vi "GetDutMAC.vi"(1 "MAC模式":string, 2 "Dut_ip":string, 3 "MAC跳数":string, 4 "Client_ip":string) -> (0 "输出MAC":string)   [LabVIEW 2014]
panel:
  out "字符串":string
  out "布尔":bool=TRUE
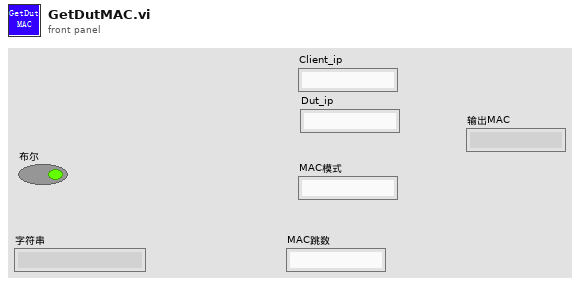
[diagram p1: front panel]
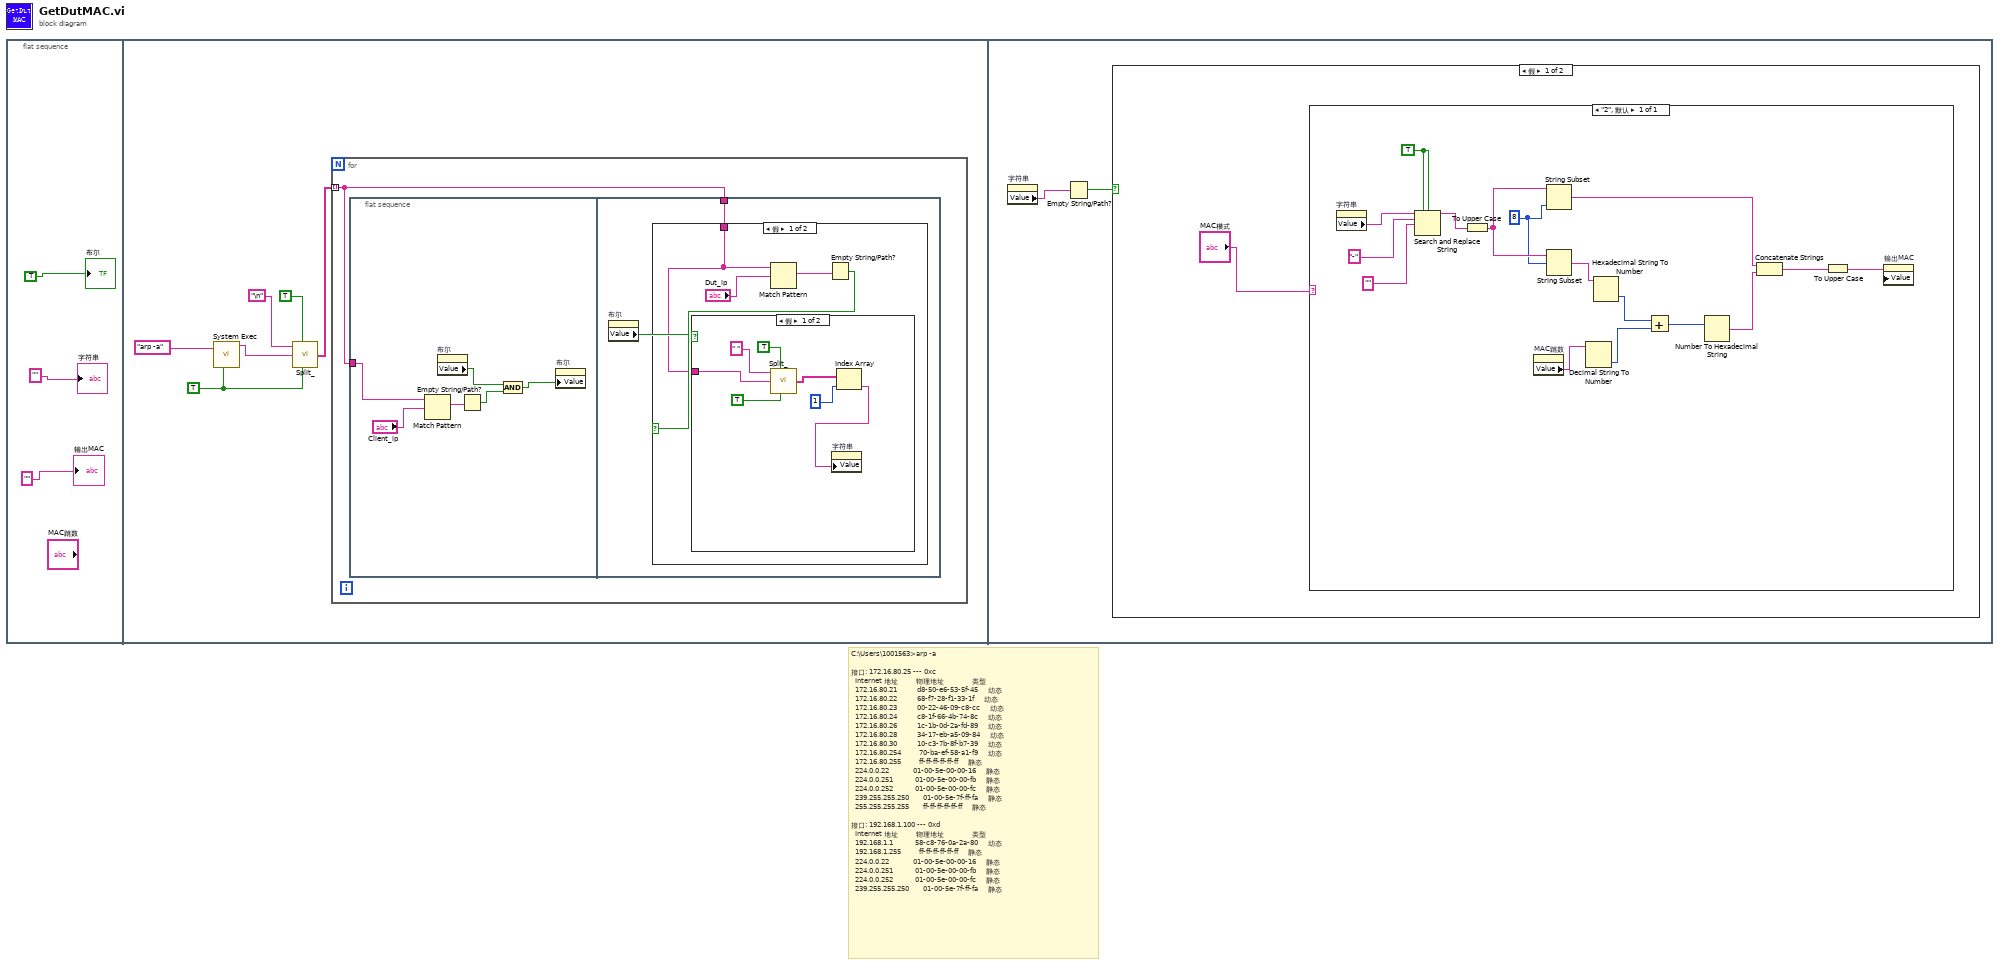
[diagram p0: block diagram]
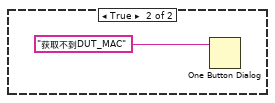
[diagram p4: hidden frame]
diagram:
  # "C:\\Users\\1001563>arp -a\n\n接口: 172.16.80.25 --- 0xc\n  Internet 地址         物理地址              类型\n  172.16.80.21          d8-50-e6-53-5f-45     动态\n  172.16.80.22          68-f7-28-f1-33-1f     动态\n  172.16.80.23          00-22-46-09-c8-cc     动态\n  172.16.80.24          c8-1f-66-4b-74-8c     动态\n  172.16.80.26          1c-1b-0d-2a-fd-89     动态\n  172.16.80.28          34-17-eb-a5-09-84     动态\n  172.16.80.30          10-c3-7b-8f-b7-39     动态\n  172.16.80.254         70-ba-ef-58-a1-f9     动态\n  172.16.80.255         ff-ff-ff-ff-ff-ff     静态\n  224.0.0.22            01-00-5e-00-00-16     静态\n  224.0.0.251           01-00-5e-00-00-fb     静态\n  224.0.0.252           01-00-5e-00-00-fc     静态\n  239.255.255.250       01-00-5e-7f-ff-fa     静态\n  255.255.255.255       ff-ff-ff-ff-ff-ff     静态\n\n接口: 192.168.1.100 --- 0xd\n  Internet 地址         物理地址              类型\n  192.168.1.1           58-c8-76-0a-2a-80     动态\n  192.168.1.255         ff-ff-ff-ff-ff-ff     静态\n  224.0.0.22            01-00-5e-00-00-16     静态\n  224.0.0.251           01-00-5e-00-00-fb     静态\n  224.0.0.252           01-00-5e-00-00-fc     静态\n  239.255.255.250       01-00-5e-7f-ff-fa     静态"
  n1 = flat-sequence {
    frame #0 {
      "布尔" <- TRUE
      "字符串" <- ""
      "输出MAC" <- ""
    }
    frame #1 {
      w5 = TRUE
      n2 = call <vilib>:"System Exec.vi"("run minimized? (F)"=w5, "command line"="arp -a") -> ("standard output"=w8:string)  [unwired: 6 in, 3 out]
      n3 = call "Split_.vi"("分隔字符串/字符(,)"="\n", "移除空字符串（T）"=TRUE, "字符串"=w8, "移除空白字符（T）"=w5) -> ("字符串数组"=w4:string[])  [unwired: 3 in]
      n4 = for {
        tunnel: w4 -> [w10] mode=indexing
        n5 = flat-sequence {
          tunnel: w10 -> [w16]
          tunnel: w10 -> [w17]
          frame #0 {
            n6 = Match Pattern(string=w16, regular expression="Client_ip") -> (match substring=w14:string)  [unwired: 1 in, 3 out]
            n7 = property on="布尔" class="Bool (严格)"() -> ("Value"=w12:bool)  [unwired: 2 in, 2 out]
            n8 = Empty String/Path?(string/path=w14) -> (empty?=w13:bool)
            n9 = And(x=w12, y=w13) -> (x .and. y?=w11:bool)
            n10 = property on="布尔" class="Bool (严格)"("Value"=w11) -> ()  [unwired: 2 in, 2 out]
          }
          frame #1 {
            n11 = property on="布尔" class="Bool (严格)"() -> ("Value"=w18:bool)  [unwired: 2 in, 2 out]
            n12 = case shown="假" w18 {
              tunnel: w17 -> [w19 _]
              frame False {
                n13 = Match Pattern(string=w19, regular expression="Dut_ip") -> (match substring=w21:string)  [unwired: 1 in, 3 out]
                n14 = Empty String/Path?(string/path=w21) -> (empty?=w20:bool)
                n15 = case shown="假" w20 {
                  tunnel: w19 -> [w29 _]
                  frame False {
                    n16 = call "Split_.vi"("分隔字符串/字符(,)"=" ", "移除空字符串（T）"=TRUE, "字符串"=w29, "移除空白字符（T）"=TRUE) -> ("字符串数组"=w25:string[])  [unwired: 3 in]
                    n17 = Index Array(array=w25, index=1) -> (element=w23:string)
                    n18 = property on="字符串" class="Str"("Value"=w23) -> ()  [unwired: 2 in, 2 out]
                  }
                  frame True {
                  }
                }
              }
              frame True {
              }
            }
          }
        }
      }
    }
    frame #2 {
      n19 = property on="字符串" class="Str"() -> ("Value"=w31:string)  [unwired: 2 in, 2 out]
      n20 = Empty String/Path?(string/path=w31) -> (empty?=w30:bool)
      n21 = case shown="假" w30 {
        frame False {
          n22 = case shown="\"2\", 默认" "MAC模式" {
            frame "2", Default {
              w37 = 8
              w45 = TRUE
              n23 = property on="字符串" class="Str"() -> ("Value"=w48:string)  [unwired: 2 in, 2 out]
              n24 = Search and Replace String(replace all?=w45, case sensitive?=w45, input string=w48, search string="-", replace string="") -> (result string=w44:string)  [unwired: 3 in, 3 out]
              n25 = To Upper Case(1:w44) -> (0:w38:string)
              n26 = property on="MAC跳数" class="Str"() -> ("Value"=w42:string)  [unwired: 2 in, 2 out]
              n27 = String Subset(string=w38, length (rest)=w37) -> (substring=w35:string)  [unwired: 1 in]
              n28 = String Subset(string=w38, offset (0)=w37) -> (substring=w36:string)  [unwired: 1 in]
              n29 = Decimal String To Number(string=w42) -> (number=w41:i32)  [unwired: 2 in, 1 out]
              n30 = Hexadecimal String To Number(string=w36) -> (number=w43:u32)  [unwired: 2 in, 1 out]
              n31 = Add(x=w43, y=w41) -> (x+y=w40:u32)
              n32 = Number To Hexadecimal String(2:w40) -> (0:w34:string)  [unwired: 1 in]
              n33 = Concatenate Strings(w35, w34) -> (w33:string)
              n34 = To Upper Case(1:w33) -> (0:w39:string)
              n35 = property on="输出MAC" class="Str"("Value"=w39) -> ()  [unwired: 2 in, 2 out]
            }
          }
        }
        frame True {
          n36 = One Button Dialog(message="获取不到DUT_MAC") -> ()  [unwired: 1 in, 1 out]
        }
      }
    }
  }
